vi "Move.vi"(8 "error in (no error)":errorcluster) -> (0 "error out":errorcluster)   [LabVIEW 2016, in "SeqProcessor.lvlib"]
uses:
  SeqProcessor.lvlib
  controls/StepType.ctl
  controls/StepIndex.ctl
  controls/Step.ctl
  controls/NormalStep.ctl
  controls/StepAction.ctl
  controls/StepResult.ctl
  controls/StepStatus.ctl
  controls/JumpStep.ctl
panel:
  in  "Seq":T2(array[cluster])=[{"Type"=enum."Parallel", "Step"=[{"Action"="SeqAbsolutePosition", "Process"="Travel", "Jump"=0, "Data"="RunTimePara.TravelTargetPosition", "Condition"=FALSE}, {"Action"="SeqAbsolutePosition", "Process"="Lift", "Jump"=0, "Data"="RunTimePara.LiftTargetPosition", "Condition"=FALSE}, {"Action"="SeqAbsolutePosition", "Process"="Rotate", "Jump"=0, "Data"="RunTimePara.RotateTargetPosition", "Condition"=FALSE}]}]
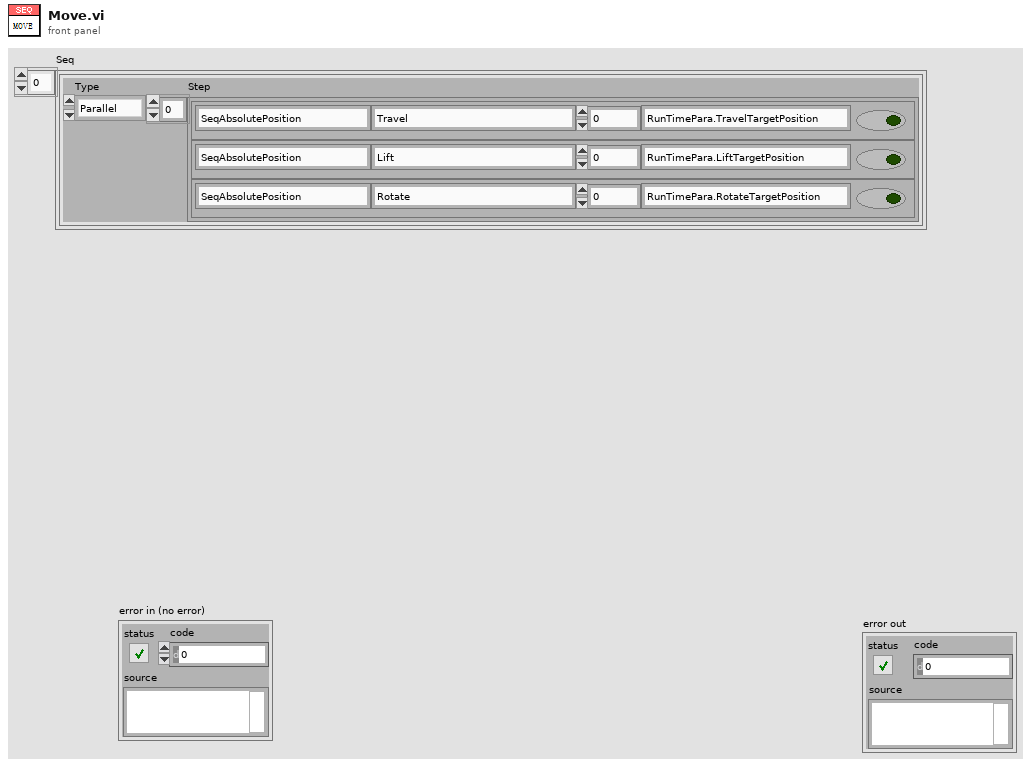
[diagram p1: front panel]
types:
  T1 = typedef "SeqProcessor.lvlib/StepType.ctl" = enum16{"Normal", "Parallel", "Conditional", "Jump"}
  T2 = cluster{"Type":T1, "Step":cluster{"Action":string, "Process":string, "Jump":i32, "Data":string, "Condition":bool}[]}[]
  T3 = typedef "SeqProcessor.lvlib/Step.ctl" = cluster{"Type":T1, "Step":variant}
  T4 = typedef "SeqProcessor.lvlib/StepIndex.ctl" = cluster{"Index1":u32, "Index2":u32}
  T5 = typedef "SeqProcessor.lvlib/StepAction.ctl" = cluster{"Action":string, "Process":string, "Data":variant, "Condition":variant}
  T6 = typedef "SeqProcessor.lvlib/NormalStep.ctl" = cluster{"Action":T5, "Result":T7}
  T7 = typedef "SeqProcessor.lvlib/StepResult.ctl" = cluster{"Status":T8, "Message":string, "Data":variant}
  T8 = typedef "SeqProcessor.lvlib/StepStatus.ctl" = enum16{"Undone", "Finish", "Error"}
  T9 = typedef "SeqProcessor.lvlib/JumpStep.ctl" = cluster{"Action":T5, "Jump":i32, "Result":T7}
  T10 = cluster{"Action":string, "Process":string, "Jump":i32, "Data":string, "Condition":bool}[]
  T11 = cluster{"Action":string, "Process":string, "Jump":i32, "Data":string, "Condition":bool}
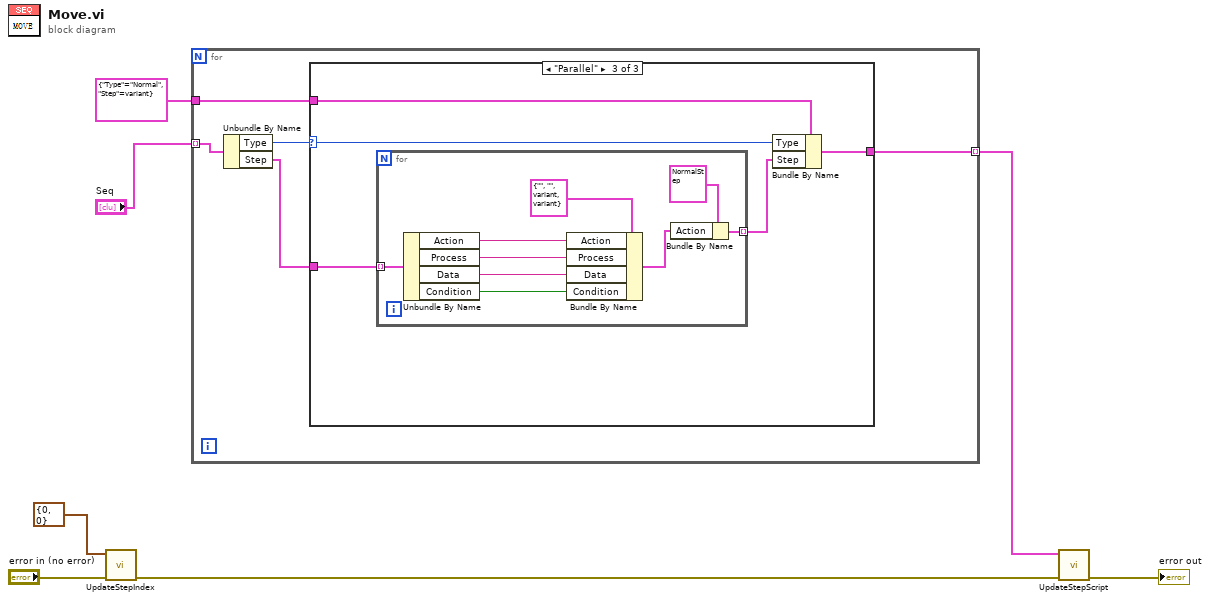
[diagram p0: block diagram]
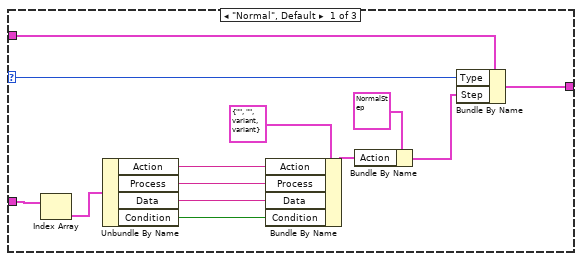
[diagram p2: hidden frame]
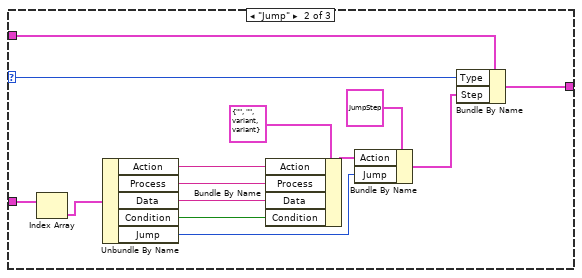
[diagram p3: hidden frame]
diagram:
  n1 = call "UpdateStepIndex.vi"("error in (no error)"="error in (no error)", "Index"=T4 {"Index1"=0, "Index2"=0}) -> ("error out"=w6:errorcluster)  [unwired: 9 in]
  n2 = for {
    tunnel: T3 {"Type"=enum."Normal", "Step"=variant} ("Step") -> [w11]
    tunnel: "Seq" -> [w9] mode=indexing
    tunnel: [w10] -> w1 mode=indexing
    n3 = Unbundle By Name(w9) -> ("Type"=w12:T1, "Step"=w8:T10)
    n4 = case shown="\"Parallel\"" w12 {
      selector: w12 -> [w23 w38 w42]
      tunnel: w8 -> [w14 w27 w44]
      tunnel: w11 -> [w24 w39 w43]
      tunnel: [w22 w37 w41] -> w10
      frame "Normal", Default {
        n5 = Index Array(array=w14) -> (element=w13:T11)  [unwired: 1 in]
        n6 = Unbundle By Name(w13) -> ("Action"=w18:string, "Process"=w17:string, "Data"=w16:string, "Condition"=w15:bool)
        n7 = Bundle By Name(cluster=T5 {"Action"="", "Process"="", "Data"=variant, "Condition"=variant} ("Action"), "Action"=w18, "Process"=w17, "Data"=w16, "Condition"=w15) -> (w19:T5)
        n8 = Bundle By Name(cluster=T6 {"Action"={"Action"="", "Process"="", "Data"=variant, "Condition"=variant(bool FALSE)}, "Result"={"Status"=enum."Undone", "Message"="", "Data"=variant}} ("NormalStep"), "Action"=w19) -> (w21:T6)
        n9 = Bundle By Name(cluster=w24, "Type"=w23, "Step"=w21) -> (w22:T3)
      }
      frame "Jump" {
        n10 = Index Array(array=w27) -> (element=w26:T11)  [unwired: 1 in]
        n11 = Unbundle By Name(w26) -> ("Action"=w33:string, "Process"=w32:string, "Data"=w31:string, "Condition"=w30:bool, "Jump"=w28:i32)
        n12 = Bundle By Name(cluster=T5 {"Action"="", "Process"="", "Data"=variant, "Condition"=variant} ("Action"), "Action"=w33, "Process"=w32, "Data"=w31, "Condition"=w30) -> (w34:T5)
        n13 = Bundle By Name(cluster=T9 {"Action"={"Action"="", "Process"="", "Data"=variant, "Condition"=variant(bool FALSE)}, "Jump"=0, "Result"={"Status"=enum."Undone", "Message"="", "Data"=variant}} ("JumplStep"), "Action"=w34, "Jump"=w28) -> (w36:T9)
        n14 = Bundle By Name(cluster=w39, "Type"=w38, "Step"=w36) -> (w37:T3)
      }
      frame "Parallel" {
        n15 = for {
          tunnel: w44 -> [w53] mode=indexing
          tunnel: [w45] -> w40 mode=indexing
          n16 = Unbundle By Name(w53) -> ("Action"=w51:string, "Process"=w50:string, "Data"=w49:string, "Condition"=w48:bool)
          n17 = Bundle By Name(cluster=T5 {"Action"="", "Process"="", "Data"=variant, "Condition"=variant} ("Action"), "Action"=w51, "Process"=w50, "Data"=w49, "Condition"=w48) -> (w46:T5)
          n18 = Bundle By Name(cluster=T6 {"Action"={"Action"="", "Process"="", "Data"=variant, "Condition"=variant(bool FALSE)}, "Result"={"Status"=enum."Undone", "Message"="", "Data"=variant}} ("NormalStep"), "Action"=w46) -> (w45:T6)
        }
        n19 = Bundle By Name(cluster=w43, "Type"=w42, "Step"=w40) -> (w41:T3)
      }
    }
  }
  n20 = call "UpdateStepScript.vi"("error in (no error)"=w6, "StepScript"=w1) -> ("error out"=→"error out":errorcluster)  [unwired: 9 in]
